vi "Execute.vi"(8 "error in (no error)":errorcluster, 11 "UDP_Receiver in":refnum<class "UDP_Receiver.lvclass">) -> (0 "error out":errorcluster, 3 "UDP_Receiver out":refnum<class "UDP_Receiver.lvclass">)   [LabVIEW 2021, in "UDP_Receiver.lvclass"]
uses:
  UDP_Receiver.lvclass
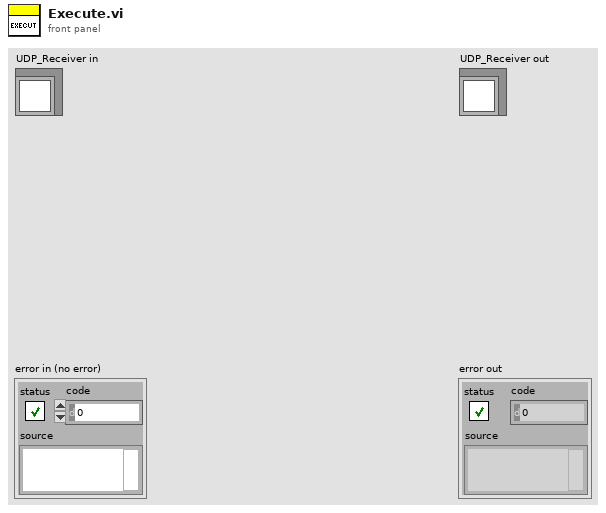
[diagram p1: front panel]
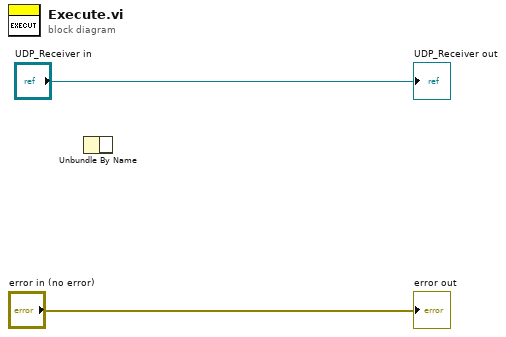
[diagram p0: block diagram]
diagram:
  n1 = Unbundle By Name() -> ()  [unwired: 1 in, 1 out]
  "error out" <- "error in (no error)"
  "UDP_Receiver out" <- "UDP_Receiver in"
